vi "Append Block.vi"(10 "block in":u8[](array[numeric]) format="%02x", 11 "Hash Function in":refnum<class "NI_SHA-256.lvclass">) -> (3 "Hash Function out":refnum<class "NI_SHA-256.lvclass">)   [LabVIEW 2020, in "NI_SHA-256.lvclass"]
uses:
  <vilib>/security/Message Digest/SHA-2/SHA-256/NI_SHA-256.lvclass
  <vilib>/security/Message Digest/SHA-2/SHA-256/NI_SHA-256.lvclass/NI_SHA-256.ctl
  <vilib>/Bit Manipulation/wrappers/Network-Order Bytes To Words/Network-Order Bytes To Words U32.vi
  <vilib>/Bit Manipulation/NI_Bit Manipulation.lvlib
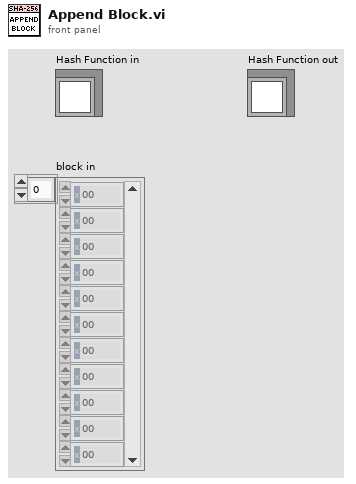
[diagram p1: front panel]
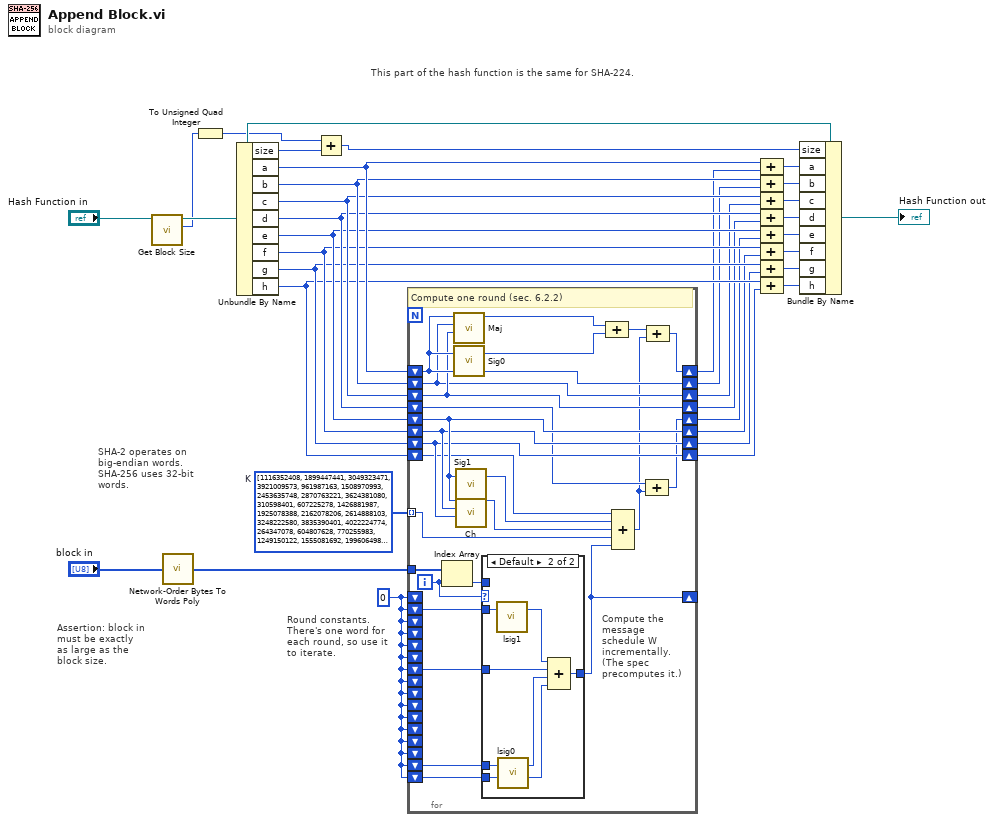
[diagram p0: block diagram]
diagram:
  w1 = u32 0
  w10 = u32[] [1116352408, 1899447441, 3049323471, 3921009573, 961987163, 1508970993, 2453635748, 2870763221, 3624381080, 310598401, 607225278, 1426881987, 1925078388, 2162078206, 2614888103, 3248222580, 3835390401, 4022224774, 264347078, 604807628, 770255983, 1249150122, 1555081692, 1996064986, 2554220882, 2821834349, 2952996808, 3210313671, 3336571891, 3584528711, 113926993, 338241895, 666307205, 773529912, 1294757372, 1396182291, 1695183700, 1986661051, 2177026350, 2456956037, 2730485921, 2820302411, 3259730800, 3345764771, 3516065817, 3600352804, 4094571909, 275423344, 430227734, 506948616, 659060556, 883997877, 958139571, 1322822218, 1537002063, 1747873779, 1955562222, 2024104815, 2227730452, 2361852424, 2428436474, 2756734187, 3204031479, 3329325298]  # K
  # "This part of the hash function is the same for SHA-224."
  # "Round constants. There's one word for each round, so use it to iterate."
  # "Assertion: block in must be exactly as large as the block size."
  # "SHA-2 operates on big-endian words. SHA-256 uses 32-bit words."
  n1 = call <vilib>:"Get Block Size.vi"("Hash Function in"="Hash Function in") -> ("block size (bytes)"=w30:i32, "Hash Function out"=w31:refnum<class "NI_SHA-256.lvclass">)  [unwired: 9 in]
  n2 = call-poly <vilib>:"Network-Order Bytes To Words Poly.vi"("bytes in"="block in") -> ("words out"=w33:u32[])
  n3 = To Unsigned Quad Integer(1:w30) -> (0:w29:u64)
  n4 = Unbundle By Name(w31) -> ("size"=w28:u64, "a"=w18:u32, "b"=w17:u32, "c"=w16:u32, "d"=w15:u32, "e"=w14:u32, "f"=w13:u32, "g"=w12:u32, "h"=w11:u32)
  n5 = Add(x=w29, y=w28) -> (x+y=w27:u64)
  n6 = for {
    shift-right: [w44] -> w9
    shift-left: w18 -> [w51]
    shift-right: [w51] -> w8
    shift-left: w17 -> [w49]
    shift-right: [w49] -> w7
    shift-left: w16 -> [w50]
    shift-right: [w50] -> w6
    shift-left: w15 -> [w53]
    shift-right: [w52] -> w5
    shift-left: w14 -> [w60]
    shift-right: [w60] -> w4
    shift-left: w13 -> [w59]
    shift-right: [w59] -> w3
    shift-left: w12 -> [w58]
    shift-right: [w58] -> w2
    shift-left: w11 -> [w57]
    tunnel: w10 -> [w54] mode=indexing
    tunnel: w33 -> [w43]
    shift-right: [w36] -> _
    shift-left: w1 -> [_]
    shift-left: w1 -> [w40]
    shift-left: w1 -> [_]
    shift-left: w1 -> [_]
    shift-left: w1 -> [_]
    shift-left: w1 -> [_]
    shift-left: w1 -> [w39]
    shift-left: w1 -> [_]
    shift-left: w1 -> [_]
    shift-left: w1 -> [_]
    shift-left: w1 -> [_]
    shift-left: w1 -> [_]
    shift-left: w1 -> [_]
    shift-left: w1 -> [_]
    shift-left: w1 -> [w38]
    shift-left: w1 -> [w37]
    i -> [w42]
    # "Compute the message schedule W incrementally. (The spec precomputes it.)"
    # "Compute one round (sec. 6.2.2)"
    n7 = Index Array(array=w43, index=w42) -> (element=w41:u32)
    n8 = call <vilib>:"Maj.vi"("z"=w50, "y"=w49, "x"=w51) -> ("Maj"=w48:u32)  [unwired: 8 in]
    n9 = call <vilib>:"Sig0.vi"("x"=w51) -> ("Sig0"=w47:u32)  [unwired: 2 in]
    n10 = call <vilib>:"Sig1.vi"("x"=w60) -> ("Sig1"=w56:u32)  [unwired: 2 in]
    n11 = call <vilib>:"Ch.vi"("z"=w58, "y"=w59, "x"=w60) -> ("Ch"=w55:u32)  [unwired: 8 in]
    n12 = case shown="Default" w42 {
      tunnel: w40 -> [_ w68]
      tunnel: w39 -> [_ w66]
      tunnel: w38 -> [_ w65]
      tunnel: w37 -> [_ w63]
      tunnel: [w61 w62] -> w36
      tunnel: w41 -> [w61 _]
      frame 0..15 {
      }
      frame Default {
        n13 = call <vilib>:"lsig1.vi"("x"=w68) -> ("lsig1"=w67:u32)  [unwired: 2 in]
        n14 = call <vilib>:"lsig0.vi"("x"=w65) -> ("lsig0"=w64:u32)  [unwired: 2 in]
        n15 = Compound Arithmetic op=ADD(w67, w66, w64, w63) -> (w62:u32)
      }
    }
    n16 = Compound Arithmetic op=ADD(w48, w47) -> (w46:u32)
    n17 = Compound Arithmetic op=ADD(w57, w56, w55, w54, w36) -> (w45:u32)
    n18 = Compound Arithmetic op=ADD(w53, w45) -> (w52:u32)
    n19 = Compound Arithmetic op=ADD(w46, w45) -> (w44:u32)
  }
  n20 = Compound Arithmetic op=ADD(w18, w9) -> (w26:u32)
  n21 = Compound Arithmetic op=ADD(w17, w8) -> (w25:u32)
  n22 = Compound Arithmetic op=ADD(w16, w7) -> (w24:u32)
  n23 = Compound Arithmetic op=ADD(w15, w6) -> (w23:u32)
  n24 = Compound Arithmetic op=ADD(w14, w5) -> (w22:u32)
  n25 = Compound Arithmetic op=ADD(w13, w4) -> (w21:u32)
  n26 = Compound Arithmetic op=ADD(w12, w3) -> (w20:u32)
  n27 = Compound Arithmetic op=ADD(w11, w2) -> (w19:u32)
  n28 = Bundle By Name(cluster=w31, "size"=w27, "a"=w26, "b"=w25, "c"=w24, "d"=w23, "e"=w22, "f"=w21, "g"=w20, "h"=w19) -> (→"Hash Function out":refnum<class "NI_SHA-256.lvclass">)
